vi "Get Alignment.vi"(2 "shared":refnum<class "niUSRP Rx Core v1 FPGA.lvclass">=refnum) -> (4 "align":refnum<class "niVST Shared Alignment v1 FPGA.lvclass">)   [LabVIEW 2023]
doc: "this VI is an accessor for Timing Information that contains the shared resource for Time-Keeping used by Alginment."
uses:
  <instrlib>/niUSRP/Reference FPGA/Rx Core/niUSRP Rx Core v1 FPGA.lvclass
  <instrlib>/niVST/Reference FPGA/FPGA/Shared/v1/Alignment/niVST Shared Alignment v1 FPGA.lvclass
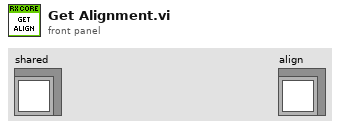
[diagram p1: front panel]
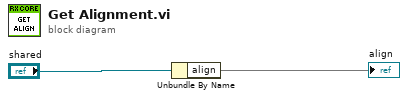
[diagram p0: block diagram]
diagram:
  n1 = Unbundle By Name("shared") -> ("align"=→"align")
